vi "createModuleManager.vi"(8 "error in (no error)":errorcluster, 10 "sensorName":string, 11 "path in":path=path "C:/dev/Hexagon-VTD-Custom-Device/Libraries/VC.dll") -> (0 "error out":errorcluster, 3 "mmHandle":u64)   [LabVIEW 2023, in "MM.lvlib"]
uses:
  MM.lvlib
  RDB/RDB.lvlib
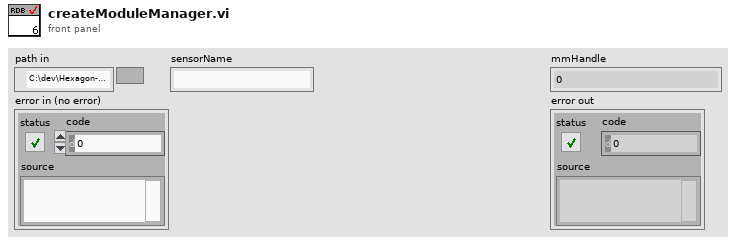
[diagram p1: front panel]
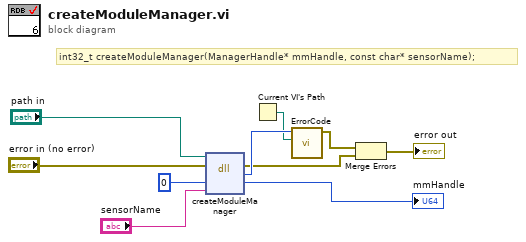
[diagram p0: block diagram]
diagram:
  # "int32_t createModuleManager(ManagerHandle* mmHandle, const char* sensorName);"
  n1 = dll-call lib="C:/dev/Hexagon-VTD-Custom-Device/Libraries/libMM.dll" fn="createModuleManager"(path in="path in", error in="error in (no error)", "mmHandle"=u64 0, "sensorName"="sensorName") -> (error out=w4:errorcluster, "return type"=w6:i32, "mmHandle"=→"mmHandle":u64)  [unwired: 2 in, 1 out]
  n2 = Current VI's Path() -> (path=w2:path)
  n3 = call "ErrorCode.vi"("parent VI path"=w2, "return type"=w6) -> ("error out"=w5:errorcluster)  [unwired: 9 in]
  n4 = Merge Errors(w5, w4) -> (→"error out":errorcluster)
